vi "ArrStrToSpreadString.vi"(10 "구분 문자":string, 11 "array str in":string[](array[string])) -> (3 "result":string caption="화이트 스페이스가 제거된 문자열")   [LabVIEW 2018, in "Library-DataConvert.lvlib"]
uses:
  Library-DataConvert.lvlib
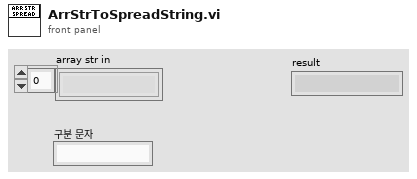
[diagram p1: front panel]
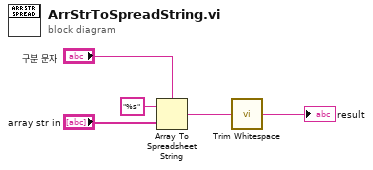
[diagram p0: block diagram]
diagram:
  n1 = Array To Spreadsheet String(delimiter (Tab)="구분 문자", array="array str in", 3:"%s" ("포맷 문자열")) -> (spreadsheet string=w2:string)
  n2 = call <vilib>:"Trim Whitespace.vi"("string"=w2) -> ("trimmed string"=→"result":string)  [unwired: 1 in]
